vi "QueueTemp.vi"(6 "Override Build\nFile Write":bool, 8 "Save Data":bool, 9 "Data In":dbl[](array[numeric]), 10 "Saving Cluster":T1, 11 "Cluster":T2) -> (2 "Number in Queue":i32, 3 "queue out":refnum<queue>)   [LabVIEW 2017]
uses:
  <vilib>/Analysis/baseanly.llb/Mean (DBL).vi
  <vilib>/Analysis/NI_AALBase.lvlib
panel:
  in  "Steady Indicator":bool=TRUE
  out "Raw Data Array":dbl[][](array[numeric])
  out "pre-arranged":dbl[][](array[numeric])
  out "Array of Averages for Build Sheet":dbl[](array[numeric])
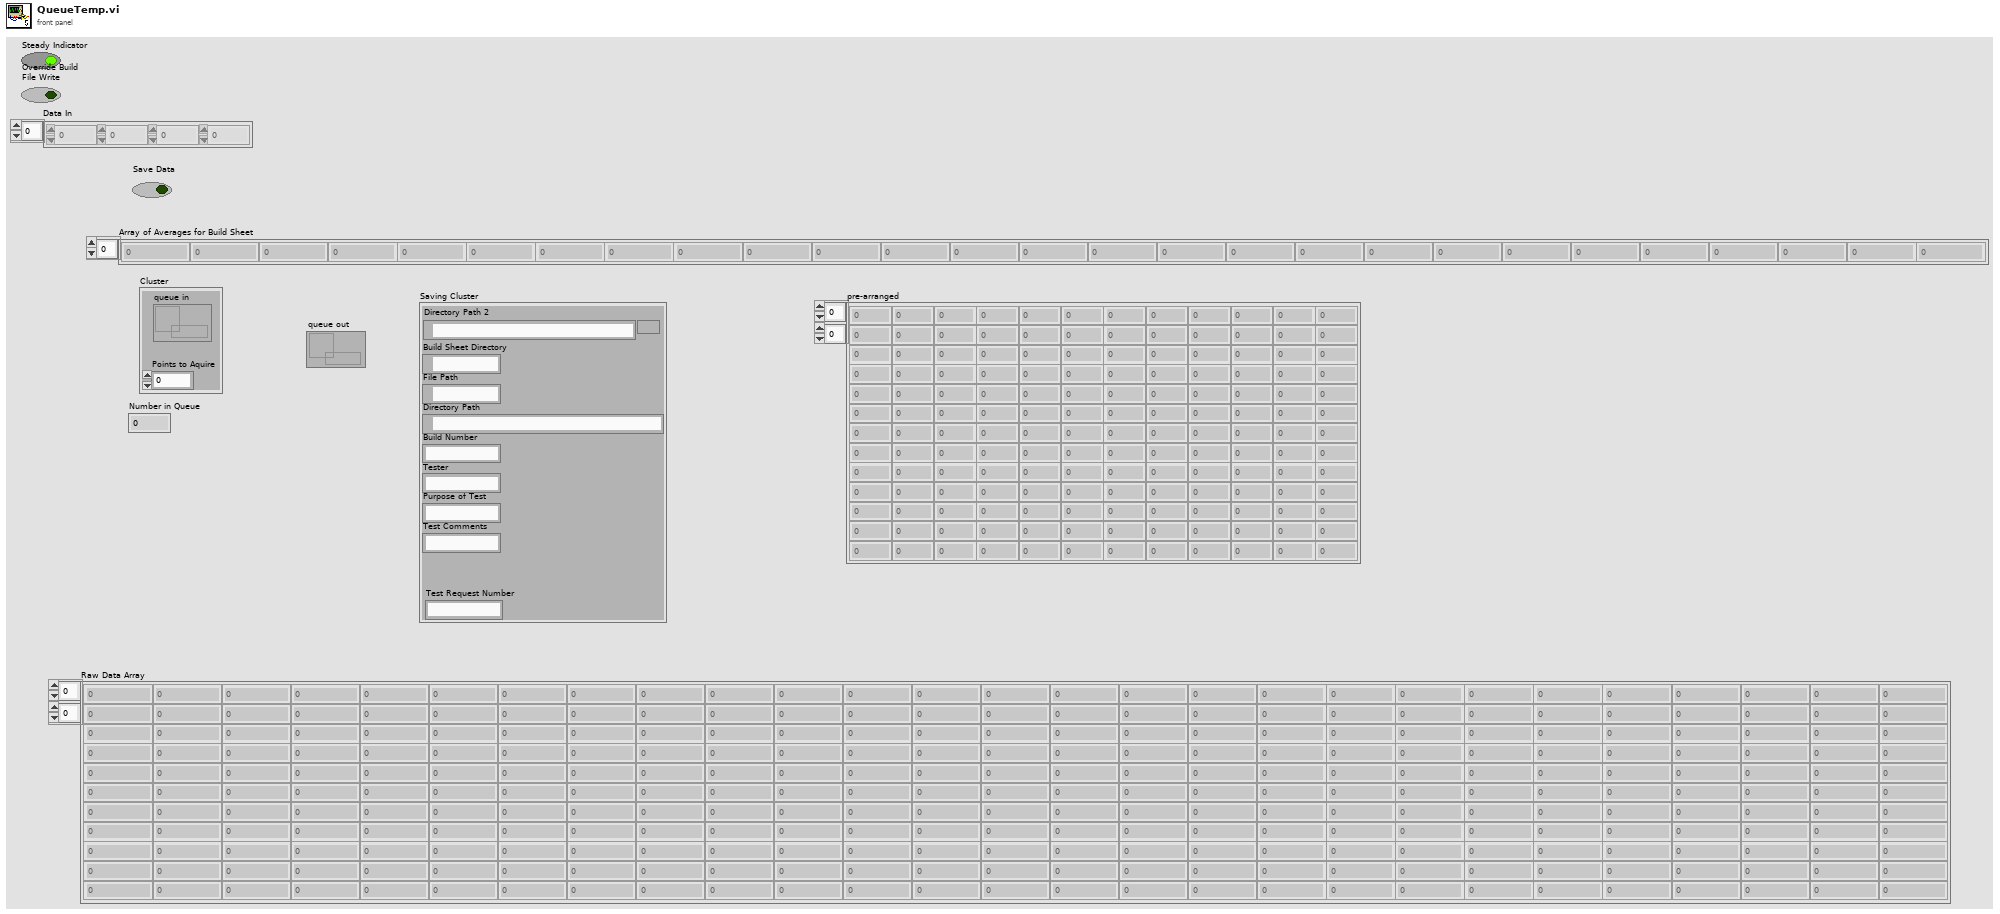
[diagram p1: front panel]
types:
  T1 = cluster{"Build Sheet Directory":path, "File Path":path, "Directory Path":path, "Build Number":string, "Tester":string, "Purpose of Test":string, "Test Comments ":string, "Test Request Number":string, "Directory Path 2":path}
  T2 = cluster{"queue in":refnum<queue>, "Points to Aquire":i32}
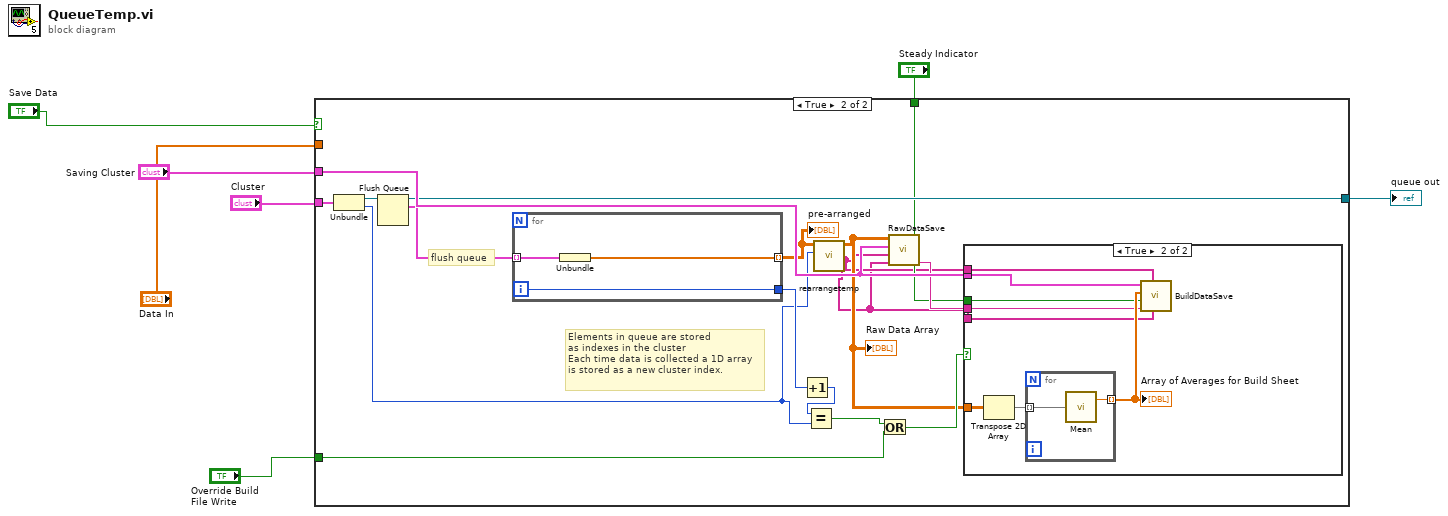
[diagram p0: block diagram]
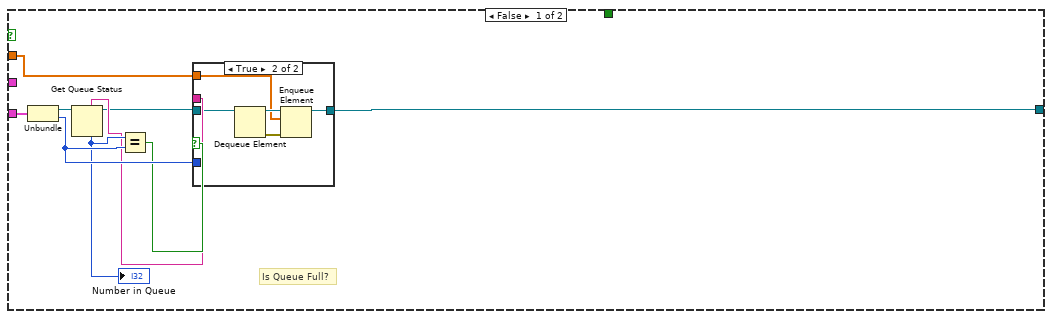
[diagram p2: hidden frame]
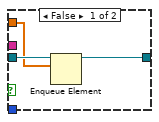
[diagram p3: hidden frame]
diagram:
  n1 = case shown="True" "Save Data" {
    tunnel: "Cluster" -> [w15 w41]
    tunnel: "Saving Cluster" -> [_ w39]
    tunnel: [w9 w38] -> w5
    tunnel: "Steady Indicator" -> [_ w35]
    tunnel: "Override Build\nFile Write" -> [_ w32]
    tunnel: "Data In" -> [w10 _]
    frame False {
      # "Is Queue Full?"
      n2 = Unbundle(w15) -> ("queue in"=w16:refnum<queue>, "Points to Aquire"=w14:i32)
      n3 = Get Queue Status(queue=w16) -> (queue out=w8:refnum<queue>, queue name=w11:string, # elements in queue=w13:i32)  [unwired: 1 in, 6 out]
      "Number in Queue" <- w13
      n4 = Equal?(x=w13, y=w14) -> (x = y?=w12:bool)
      n5 = case shown="True" w12 {
        tunnel: w14 -> [_ _]
        tunnel: w11 -> [_ _]
        tunnel: [w19 w22] -> w9
        tunnel: w8 -> [w18 w21]
        tunnel: w10 -> [w17 w20]
        frame False {
          n6 = Enqueue Element(queue=w18, element=w17) -> (queue out=w19:refnum<queue>)  [unwired: 1 in, 3 out]
        }
        frame True {
          n7 = Dequeue Element(queue=w21) -> (queue out=w24:refnum<queue>, error out=w23:errorcluster)  [unwired: 1 in, 3 out]
          n8 = Enqueue Element(queue=w24, element=w20, error in (no error)=w23) -> (queue out=w22:refnum<queue>)  [unwired: 3 out]
        }
      }
    }
    frame True {
      # "Elements in queue are stored\nas indexes in the cluster\nEach time data is collected a 1D array\nis stored as a new cluster index."
      # "flush queue"
      n9 = Unbundle(w41) -> ("queue in"=w40:refnum<queue>, "Points to Aquire"=w29:i32)
      n10 = Flush Queue(queue=w40) -> (queue out=w38:refnum<queue>, remaining elements=w37:cluster{dbl[]}[])  [unwired: 1 in, 1 out]
      n11 = for {
        tunnel: [w54] -> w28 mode=indexing
        tunnel: w37 -> [w53] mode=indexing
        tunnel: [w52] -> w31
        i -> [w52]
        n12 = Unbundle(w53) -> (w54:dbl[])
      }
      "pre-arranged" <- w28
      n13 = Increment(x=w31) -> (x+1=w30:i32)
      n14 = Equal?(x=w30, y=w29) -> (x = y?=w33:bool)
      n15 = call "rearrangetemp.vi"("Points to Aquire"=w29, "Array in"=w28) -> ("units"=w25:string[], "varnames"=w26:string[], "Array out"=w27:dbl[][])  [unwired: 6 in]
      "Raw Data Array" <- w27
      n16 = Or(x=w33, y=w32) -> (x .or. y?=w34:bool)
      n17 = call "RawDataSave.vi"("units"=w25, "varnames"=w26, "Saving Cluster"=w39, "Array"=w27) -> ("raw data filename string"=w36:string)  [unwired: 7 in]
      n18 = case shown="True" w34 {
        tunnel: w39 -> [_ w49]
        tunnel: w27 -> [_ w46]
        tunnel: w36 -> [_ w45]
        tunnel: w26 -> [_ w44]
        tunnel: w25 -> [_ w43]
        tunnel: w35 -> [_ w42]
        frame False {
        }
        frame True {
          n19 = Transpose 2D Array(2D array=w46) -> (transposed array=w48:dbl[][])
          n20 = for {
            tunnel: w48 -> [w50] mode=indexing
            tunnel: [w51] -> w47 mode=indexing
            n21 = call-poly <vilib>:"Mean.vi"("X"=w50) -> ("mean"=w51:dbl)  [unwired: 1 out]
          }
          "Array of Averages for Build Sheet" <- w47
          n22 = call "BuildDataSave.vi"("units"=w43, "varnames"=w44, "raw data filename string"=w45, "Steady Indicator"=w42, "Array"=w47, "Saving Cluster"=w49) -> ()  [unwired: 6 in]
        }
      }
    }
  }
  "queue out" <- w5
